vi "Set Voltage Range.vi"(4 "Power Line Cycles (0)":i32, 7 "Voltage Range (0: 2 Volts)":u16(ring) items=["2 Volts", "20 Volts"], 8 "error in (no error)":errorcluster, 10 "Channel (1: Channel 1)":u16(ring)=1 items=["Channel 1"=1, "Channel 2"=2, "Channel 3"=3], 11 "VISA resource name":refnum<visa-resource-name>) -> (0 "error out":errorcluster, 3 "VISA resource name out":refnum<visa-resource-name>)   [LabVIEW 2018, in "Agilent U2722.lvlib"]
doc: "Configures the channel to output in source voltage mode."
uses:
  U2722 LabVIEW Instr Driver and Examples/Agilent U2722.lvlib
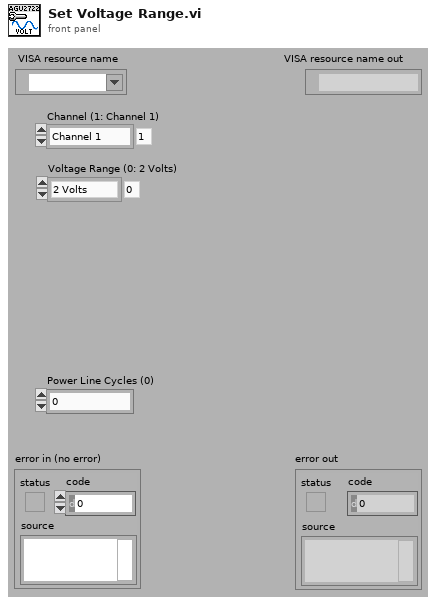
[diagram p1: front panel]
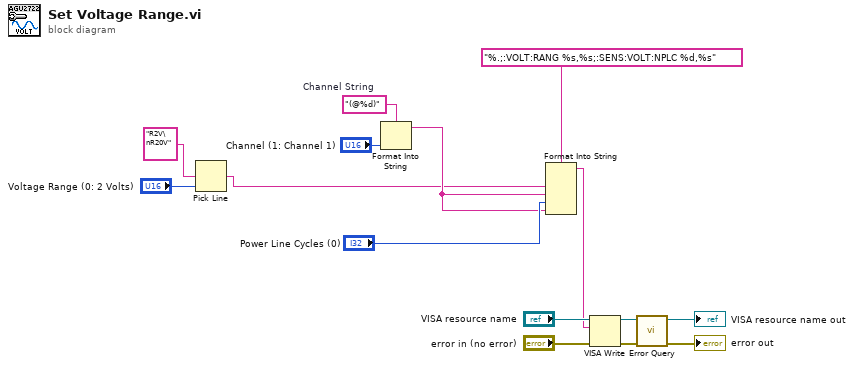
[diagram p0: block diagram]
diagram:
  w8 = "(@%d)"  # Channel String
  n1 = Pick Line(multi-line string="R2V\nR20V", line index="Voltage Range (0: 2 Volts)") -> (output string=w1:string)  [unwired: 1 in]
  n2 = Format Into String(format string=w8, "Channel (1: Channel 1)") -> (resulting string=w5:string)  [unwired: 2 in, 1 out]
  n3 = Format Into String(format string="%.;:VOLT:RANG %s,%s;:SENS:VOLT:NPLC %d,%s", w1, w5, "Power Line Cycles (0)", w5) -> (resulting string=w4:string)  [unwired: 2 in, 1 out]
  n4 = VISA Write(VISA resource name="VISA resource name", write buffer=w4, error in (no error)="error in (no error)") -> (VISA resource name out=w11:refnum<visa-resource-name>, error out=w10:errorcluster)  [unwired: 1 out]
  n5 = call "Error Query.vi"("error in (no error)"=w10, "VISA resource name"=w11) -> ("error out"=→"error out":errorcluster, "VISA resource name out"=→"VISA resource name out":refnum<visa-resource-name>)  [unwired: 6 in, 2 out]
